vi "SV Library Creator.vi"() -> ()   [LabVIEW 2013]
uses:
  <vilib>/lvdsc/process/ProcessToLib.vi
  <vilib>/lvdsc/NI_DSC.lvlib
panel:
  in  "Array":T1(array[cluster])=[{"data type"=enum."uint8", "Libs to Build"=[50, 100, 150, 200, 250, 300, 350, 400, 450, 500]}, {"data type"=enum."uint16", "Libs to Build"=[50, 100, 150, 200, 250, 300, 350, 400, 450, 500]}, {"data type"=enum."uint32", "Libs to Build"=[50, 100, 150, 200, 250, 300, 350, 400, 450, 500]}, {"data type"=enum."uint64", "Libs to Build"=[50, 100, 150, 200, 250, 300, 350, 400, 450, 500]}, {"data type"=enum."int8", "Libs to Build"=[50, 100, 150, 200, 250, 300, 350, 400, 450, 500]}, {"data type"=enum."int16", "Libs to Build"=[50, 100, 150, 200, 250, 300, 350, 400, 450, 500]}, {"data type"=enum."int32", "Libs to Build"=[50, 100, 150, 200, 250, 300, 350, 400, 450, 500]}, {"data type"=enum."int64", "Libs to Build"=[50, 100, 150, 200, 250, 300, 350, 400, 450, 500]}, {"data type"=enum."single", "Libs to Build"=[50, 100, 150, 200, 250, 300, 350, 400, 450, 500]}, {"data type"=enum."double", "Libs to Build"=[50, 100, 150, 200, 250, 300, 350, 400, 450, 500]}, {"data type"=enum."bool", "Libs to Build"=[50, 100, 150, 200, 250, 300, 350, 400, 450, 500]}, {"data type"=enum."string", "Libs to Build"=[50, 100, 150, 200, 250, 300, 350, 400, 450, 500]}]
  # "Utility for generating the necessary shared variable libraries used by the application. Requires DSC"
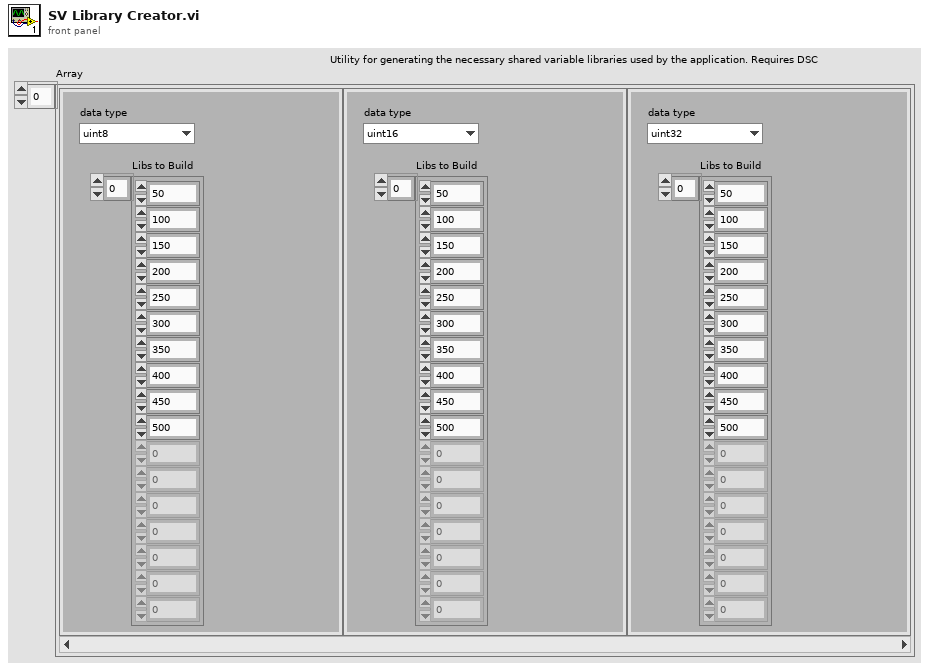
[diagram p1: front panel]
types:
  T1 = cluster{"data type":enum32{"u32BitField", "bool", "double", "string", "int8", "uint8", "int16", "uint16", "int32", "uint32", "int64", "uint64", "single", "double waveform", "int16 waveform", "array of boolean", "array of int8", "array of uint8", "array of int16", "array of uint16", "array of int32", "array of uint32", "array of int64", "array of uint64", "array of single", "array of double", "array of double waveform", "array of int16 waveform", "array of string", "variant", "timestamp", "fixed point", "custom"}, "Libs to Build":u16[]}[]
  T2 = enum32{"u32BitField", "bool", "double", "string", "int8", "uint8", "int16", "uint16", "int32", "uint32", "int64", "uint64", "single", "double waveform", "int16 waveform", "array of boolean", "array of int8", "array of uint8", "array of int16", "array of uint16", "array of int32", "array of uint32", "array of int64", "array of uint64", "array of single", "array of double", "array of double waveform", "array of int16 waveform", "array of string", "variant", "timestamp", "fixed point", "custom"}
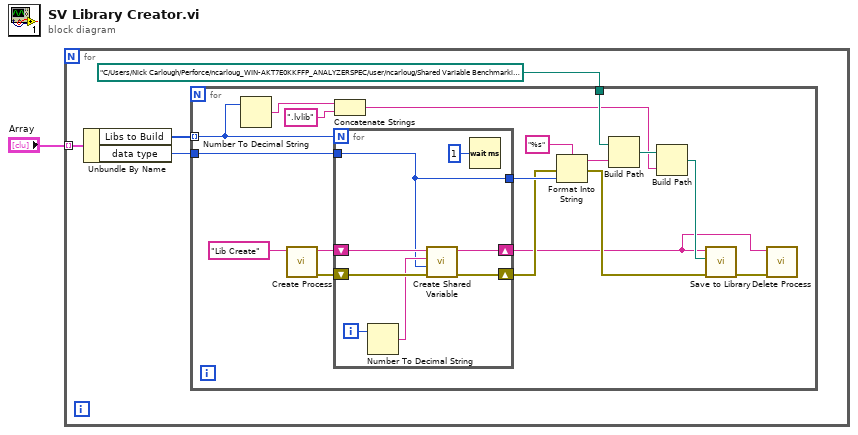
[diagram p0: block diagram]
diagram:
  n1 = for {
    tunnel: "Array" -> [w5] mode=indexing
    n2 = Unbundle By Name(w5) -> ("Libs to Build"=w4:u16[], "data type"=w3:T2)
    n3 = for {
      tunnel: w4 -> [w13] mode=indexing
      tunnel: w3 -> [w20]
      tunnel: path "C:/Users/Nick Carlough/Perforce/ncarloug_WIN-AKT7E0KKFFP_ANALYZERSPEC/user/ncarloug/Shared Variable Benchmarking Utility/builds/Windows Host/SV Libraries" -> [w19]
      n4 = Number To Decimal String(number=w13) -> (decimal integer string=w12:string)  [unwired: 1 in]
      n5 = call <vilib>:"Create Process.vi"("process name"="Lib Create") -> ("error out"=w21:errorcluster, "process name out"=w22:string)  [unwired: 9 in]
      n6 = for {
        N: w13 -> [_]
        tunnel: w20 -> [w24]
        shift-right: [w26] -> w6
        shift-left: w22 -> [w31]
        shift-right: [w25] -> w16
        shift-left: w21 -> [w30]
        tunnel: [w24] -> w18
        i -> [w29]
        n7 = Number To Decimal String(number=w29) -> (decimal integer string=w28:string)  [unwired: 1 in]
        n8 = call <vilib>:"Create Shared Variable.vi"("error in (no error)"=w30, "data type"=w24, "shared variable name"=w28, "process name"=w31) -> ("error out"=w25:errorcluster, "process name out"=w26:string)  [unwired: 5 in, 1 out]
        n9 = Wait (ms)(milliseconds to wait=u32 1) -> ()  [unwired: 1 out]
      }
      n10 = Concatenate Strings(w12, ".lvlib" ("concatenated string")) -> (w9:string)
      n11 = Format Into String(format string="%s", error in=w16, w18) -> (resulting string=w15:string, error out=w14:errorcluster)  [unwired: 1 in]
      n12 = Build Path(base path=w19, name or relative path=w15) -> (appended path=w10:path)
      n13 = Build Path(base path=w10, name or relative path=w9) -> (appended path=w8:path)
      n14 = call-poly <vilib>:"Save to Library.vi"("error in (no error)"=w14, "library path"=w8, "process"=w6) -> ("error out"=w7:errorcluster)  [unwired: 7 in, 1 out]
      n15 = call <vilib>:"Delete Process.vi"("error in (no error)"=w7, "process name"=w6) -> ()  [unwired: 9 in, 1 out]
    }
  }
